vi "Google Earth - Camera Position - Read.vi"(8 "error in":errorcluster, 11 "Refnum in":refnum<k7>) -> (0 "error out":errorcluster, 2 "Camera Position":T1, 3 "Refnum Out":refnum<k7>)   [LabVIEW 8.6]
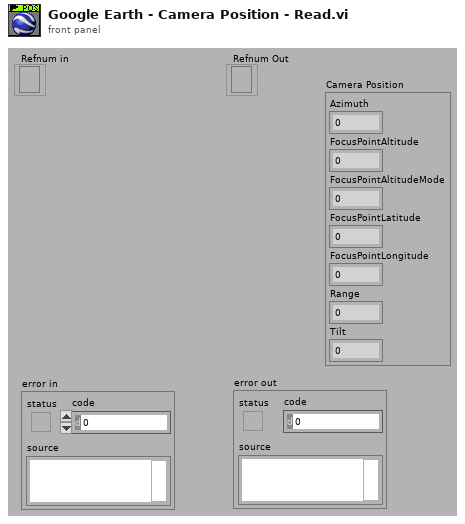
[diagram p1: front panel]
types:
  T1 = cluster{"Azimuth":dbl, "FocusPointAltitude":dbl, "FocusPointAltitudeMode":i32, "FocusPointLatitude":dbl, "FocusPointLongitude":dbl, "Range":dbl, "Tilt":dbl}
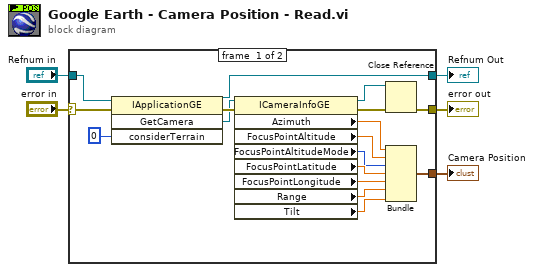
[diagram p0: block diagram]
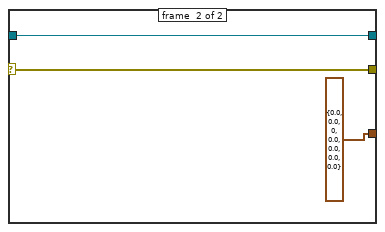
[diagram p2: hidden frame]
diagram:
  n1 = case shown="No Error" "error in" {
    selector: "error in" -> [w6 w24]
    tunnel: [w22 w24] -> w5
    tunnel: [w21 w25] -> w4
    tunnel: "Refnum in" -> [w19 w25]
    tunnel: [w7 T1 {"Azimuth"=0.0, "FocusPointAltitude"=0.0, "FocusPointAltitudeMode"=0, "FocusPointLatitude"=0.0, "FocusPointLongitude"=0.0, "Range"=0.0, "Tilt"=0.0}] -> w2
    frame #0 {
      n2 = invoke class="IApplicationGE" method="GetCamera"(reference=w19, error in=w6, "considerTerrain"=0) -> (reference out=w21:refnum<k7>, error out=w20:errorcluster, "GetCamera"=w18:refnum<k7>)  [unwired: 1 in, 1 out]
      n3 = property class="ICameraInfoGE"(reference=w18, error in=w20) -> (reference out=w15:refnum<k7>, error out=w16:errorcluster, "Azimuth"=w14:dbl, "FocusPointAltitude"=w13:dbl, "FocusPointAltitudeMode"=w10:i32, "FocusPointLatitude"=w12:dbl, "FocusPointLongitude"=w11:dbl, "Range"=w9:dbl, "Tilt"=w8:dbl)
      n4 = Close Reference(reference=w15, error in (no error)=w16) -> (error out=w22:errorcluster)
      n5 = Bundle("Azimuth"=w14, "FocusPointAltitude"=w13, "FocusPointAltitudeMode"=w10, "FocusPointLatitude"=w12, "FocusPointLongitude"=w11, "Range"=w9, "Tilt"=w8) -> (w7:T1)  [unwired: 1 in]
    }
    frame #1 {
    }
  }
  "error out" <- w5
  "Refnum Out" <- w4
  "Camera Position" <- w2
